vi "Init Log.vi"(4 "Enabled":bool=TRUE, 6 "Call Chain":bool, 7 "Level":T1=enum."Debug", 8 "error in (no error)":errorcluster, 10 "iName":string, 11 "iType":string) -> (0 "error out":errorcluster, 3 "Application Log out":refnum<class "Application Log.lvclass">)   [LabVIEW 2016, in "Stream Log.lvlib" / "Application Log.lvclass"]
doc: "--\nCopyright © 2017 Composed SystemsI All rights reserved.\n\nAuthor: Jon McBee <jon.mcbee@composed.io>\n\nThis library is provided \"AS IS\" ,WITHOUT WARRANTIES OR\nCONDITIONS OF ANY KIND, either express or implied.\n\nComposed Systems -- composed.io\n\nStream 0.0.1.1\nJon McBee - Composed Systems\nCopyright (c) 2017, Composed Systems"
uses:
  <userlib>/Composed Systems/Stream/Log/Application Log/Application Log.lvclass
  C:/Program Files (x86)/National Instruments/LabVIEW 2016/user.lib/Composed Systems/Stream/Actor/Actor Class/Ancestral Actor.lvclass
  <userlib>/Composed Systems/Stream/Log/Application Log/Log Level.ctl
  <userlib>/Composed Systems/Stream/Actor/Actor Class/Ancestral Actor.lvclass/Ancestral Actor.ctl
  <userlib>/Composed Systems/Stream/Actor/Actor Class/Ancestral Actor.lvclass
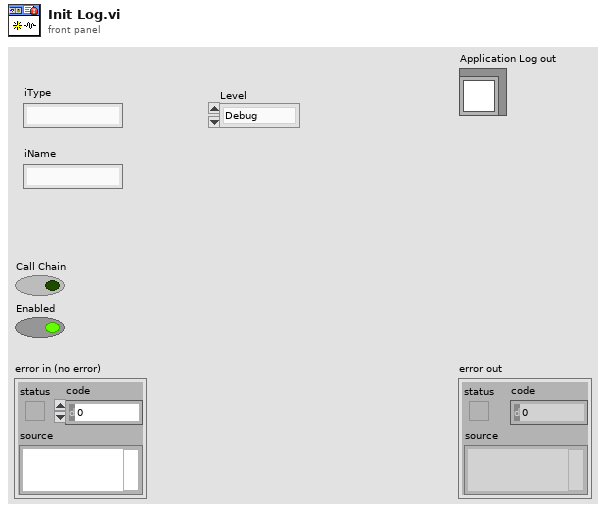
[diagram p1: front panel]
types:
  T1 = typedef "Stream Log.lvlib/Application Log.lvclass/Log Level.ctl" = enum16{"Imperative", "Major", "Minor", "Debug", "Off"}
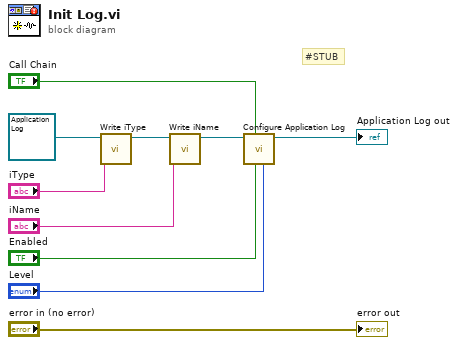
[diagram p0: block diagram]
diagram:
  # "#STUB"
  n1 = call <userlib>:"Write iType.vi"("iType"="iType", "Ancestral Actor in"=refnum<class "Application Log.lvclass"> refnum ("Application Log in")) -> ("Ancestral Actor out"=w5:refnum<class "Application Log.lvclass">)  [unwired: 8 in, 1 out]
  n2 = call <userlib>:"Write iName.vi"("iName"="iName", "Ancestral Actor in"=w5) -> ("Ancestral Actor out"=w3:refnum<class "Application Log.lvclass">)  [unwired: 8 in, 1 out]
  n3 = call-dynamic "Configure Application Log.vi"("Configuration.Level"="Level", "Configuration.Enabled"="Enabled", "Configuration.Call Chain"="Call Chain", "Application Log in"=w3) -> ("Application Log out"=→"Application Log out":refnum<class "Application Log.lvclass">)  [unwired: 6 in, 1 out]
  "error out" <- "error in (no error)"
